vi "nontime x-axis data.vi"(10 "y-axis data history":T1, 11 "x-axis data history":T1) -> (3 "XY plot":cluster{"x":dbl[], "y":dbl[]})   [LabVIEW 2021, in "RocketPlot.lvlib"]
uses:
  RocketPlot.lvlib
  TypeDefs/plot datapoint.ctl
  <userlib>/bjustice/Ring Buffer for Time Series Data Strict Accessor/SubVIs/Search for oldest time to keep.vi
  <userlib>/bjustice/Ring Buffer for Time Series Data Strict Accessor/SubVIs/Search for newest time to keep.vi
  <userlib>/bjustice/Ring Buffer for Time Series Data Strict Accessor/Ring Buffer Strict Accessor.lvlib
panel:
  out "slave":cluster{u64[], dbl[]}
  out "master":cluster{u64[], dbl[]}
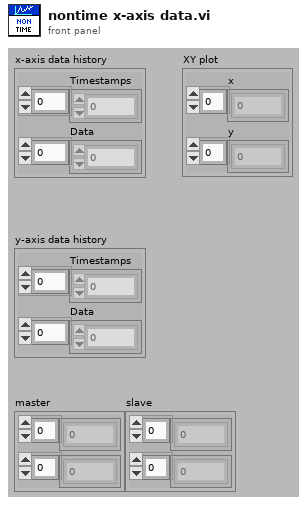
[diagram p1: front panel]
types:
  T1 = typedef "RocketPlot.lvlib/plot datapoint.ctl" = cluster{"Timestamps":u64[], "Data":dbl[]}
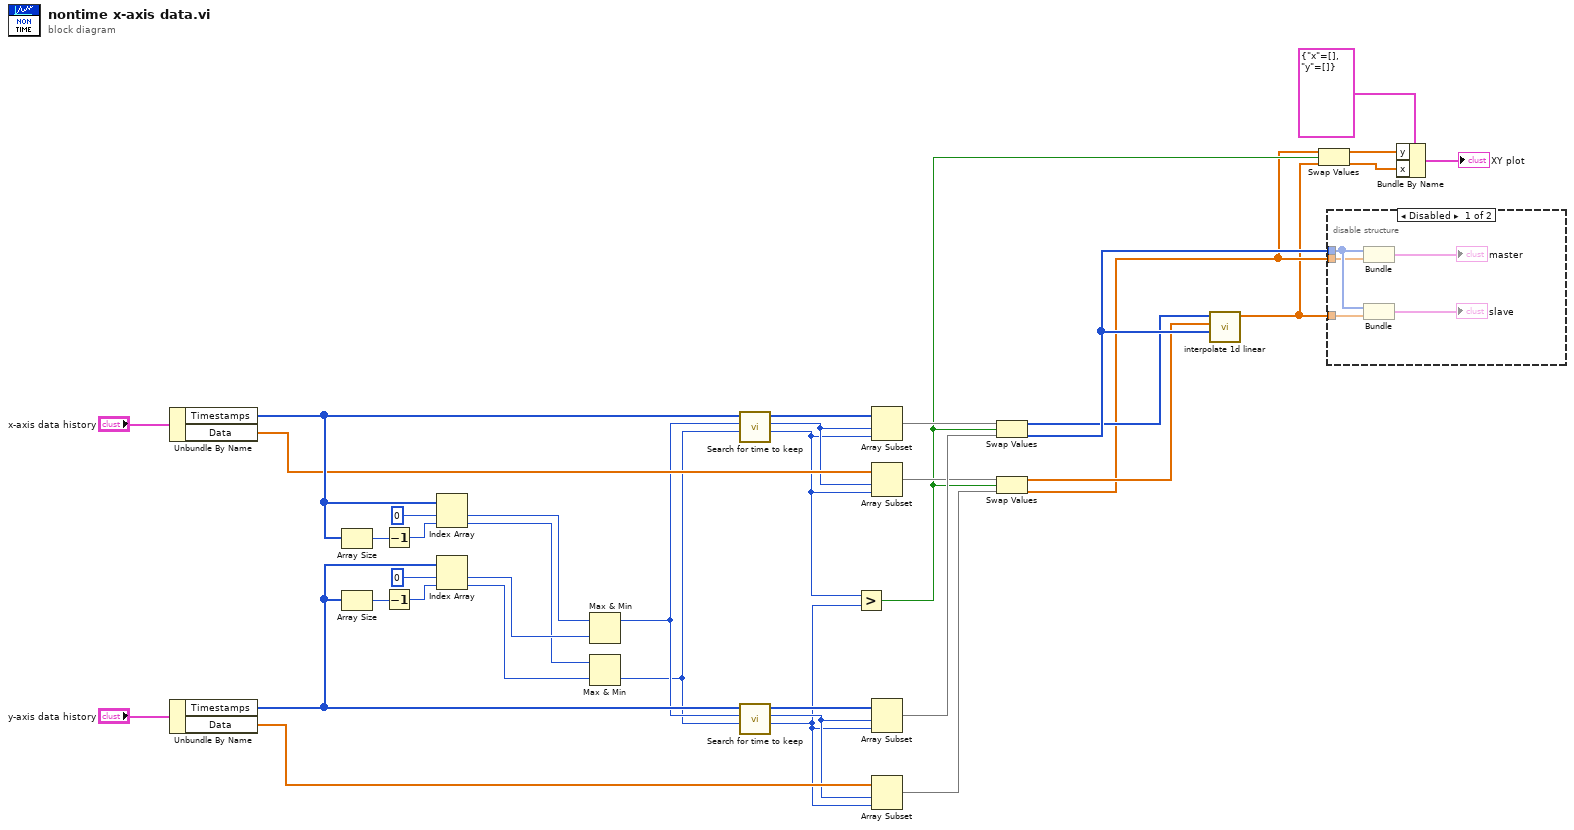
[diagram p0: block diagram]
diagram:
  n1 = Unbundle By Name("x-axis data history") -> ("Timestamps"=w32:u64[], "Data"=w24:dbl[])
  n2 = Unbundle By Name("y-axis data history") -> ("Timestamps"=w31:u64[], "Data"=w22:dbl[])
  n3 = Array Size(array=w32) -> (size(s)=w34:i32)
  n4 = Array Size(array=w31) -> (size(s)=w37:i32)
  n5 = Decrement(x=w34) -> (x-1=w35:i32)
  n6 = Decrement(x=w37) -> (x-1=w36:i32)
  n7 = Index Array(array=w32, index #1=0 ("index"), index #2=w35) -> (element #1=w30:u64, element #2=w27:u64)
  n8 = Index Array(array=w31, index #1=0 ("index"), index #2=w36) -> (element #1=w29:u64, element #2=w28:u64)
  n9 = Max & Min(x=w30, y=w29) -> (max(x,y)=w2:u64)  [unwired: 1 out]
  n10 = Max & Min(x=w27, y=w28) -> (min(x,y)=w1:u64)  [unwired: 1 out]
  n11 = call <userlib>:"Search for time to keep.vi"("newest time to keep"=w1, "oldest time to keep"=w2, "timestamps (incrementing)"=w32) -> ("length"=w20:i32, "index"=w23:i32, "timestamps (dup)"=w26:u64[])  [unwired: 6 in]
  n12 = call <userlib>:"Search for time to keep.vi"("newest time to keep"=w1, "oldest time to keep"=w2, "timestamps (incrementing)"=w31) -> ("length"=w19:i32, "index"=w21:i32, "timestamps (dup)"=w25:u64[])  [unwired: 6 in]
  n13 = Greater?(x=w20, y=w19) -> (0:w10:bool)
  n14 = Array Subset(array=w26, index=w23, length=w20) -> (w18:u64[])
  n15 = Array Subset(array=w24, index=w23, length=w20) -> (w16:dbl[])
  n16 = Array Subset(array=w25, index=w21, length=w19) -> (w17:u64[])
  n17 = Array Subset(array=w22, index=w21, length=w19) -> (w15:dbl[])
  n18 = Swap Values(12:w18, 13:w10, 14:w17) -> (1:w13:u64[], 3:w14:u64[])
  n19 = Swap Values(12:w16, 13:w10, 14:w15) -> (1:w12:dbl[], 3:w9:dbl[])
  n20 = call "interpolate 1d linear.vi"("xi"=w14, "Y"=w12, "X"=w13) -> ("yi"=w8:dbl[])  [unwired: 8 in]
  n21 = Swap Values(12:w9, 13:w10, 14:w8) -> (1:w7:dbl[], 3:w6:dbl[])
  n22 = disable-structure shown="Disabled" {
    disable-tunnel: w14 -> [w41 _]
    disable-tunnel: w9 -> [w40 _]
    disable-tunnel: w8 -> [w39 _]
    frame Disabled {
      n23 = Bundle(w41, w40) -> (→"master":cluster{u64[], dbl[]})  [unwired: 1 in]
      n24 = Bundle(w41, "yi"=w39) -> (→"slave":cluster{u64[], "yi":dbl[]})  [unwired: 1 in]
    }
    frame Enabled {
    }
  }
  n25 = Bundle By Name(cluster=cluster{"x":dbl[], "y":dbl[]} {"x"=[], "y"=[]}, "y"=w7, "x"=w6) -> (→"XY plot":cluster{"x":dbl[], "y":dbl[]})
